vi "Host-Convert-U64-to-String.vi"(11 "U64_in":u64) -> (3 "Str_out":string)   [LabVIEW 2020]
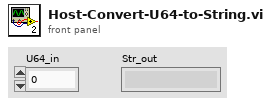
[diagram p1: front panel]
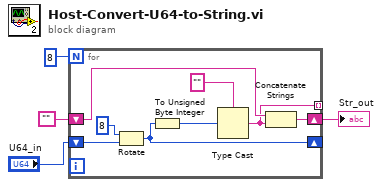
[diagram p0: block diagram]
diagram:
  n1 = for {
    N: 8 -> [_]
    shift-right: [w5] -> _
    shift-left: "U64_in" -> [w9]
    tunnel: [w6] -> _ mode=indexing
    shift-right: [w7] -> w4
    shift-left: "" -> [w8]
    n2 = Rotate(1:w9, 2:i16 8 ("y")) -> (0:w5:u64)
    n3 = To Unsigned Byte Integer(number=w5) -> (unsigned 8bit integer=w11:u8)
    n4 = Type Cast(type="", x=w11) -> (*(type *) &x=w6:string)
    n5 = Concatenate Strings(w8, w6) -> (w7:string)
  }
  "Str_out" <- w4
